vi "Robomapping.vi"(2 "Sensor View":i8[][](array[numeric]), 3 "World (mapped) in":i8[][](array[numeric]), 4 "Y":i8, 5 "X":i8) -> (0 "Sum of sensor array":i8, 1 "World (mapped) out":i8[][](array[numeric]))   [LabVIEW 2014]
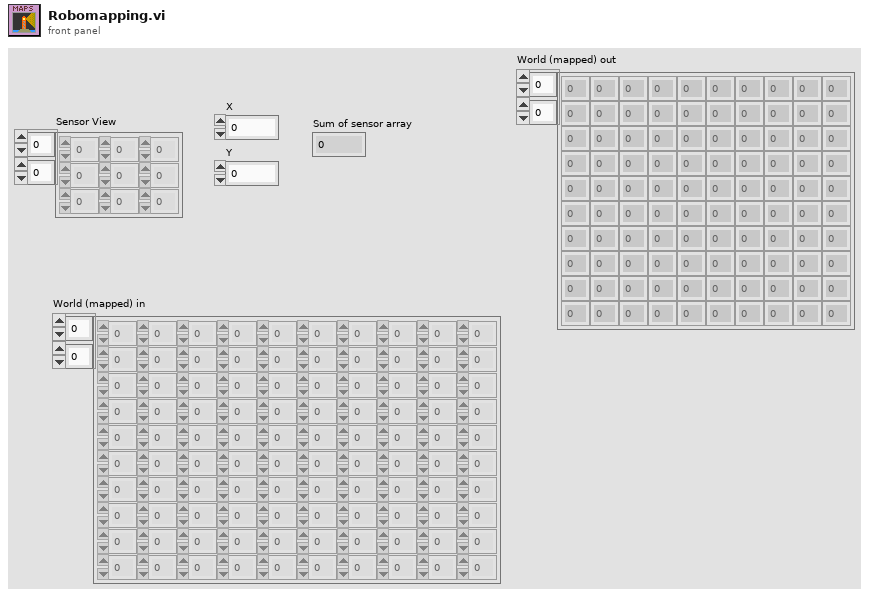
[diagram p1: front panel]
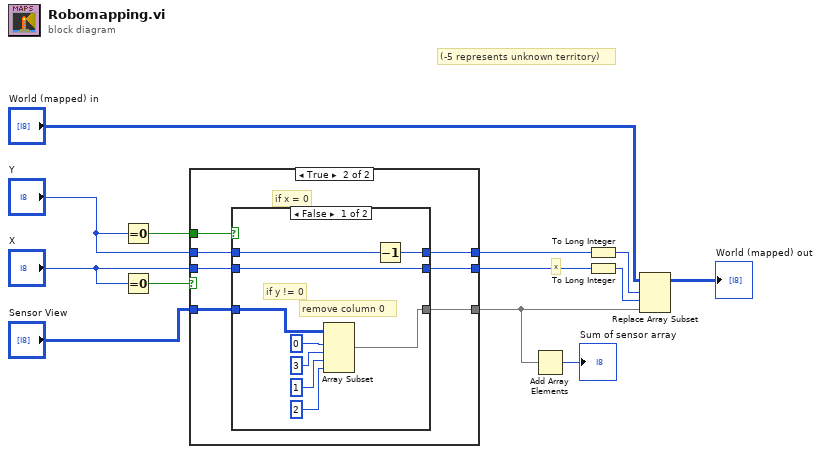
[diagram p0: block diagram]
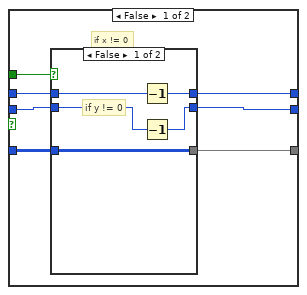
[diagram p2: hidden frame]
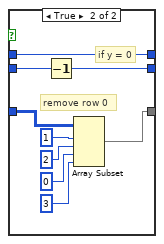
[diagram p3: hidden frame]
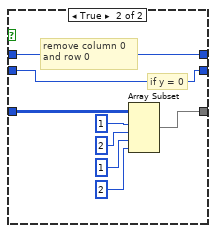
[diagram p4: hidden frame]
diagram:
  # "x"
  # "(-5 represents unknown territory)"
  n1 = Equal To 0?(x="Y") -> (x = 0?=w12:bool)
  n2 = Equal To 0?(x="X") -> (x = 0?=w13:bool)
  n3 = case shown="True" w13 {
    tunnel: "Sensor View" -> [w20 w40]
    tunnel: w12 -> [w19 w41]
    tunnel: [w16 w39] -> w2
    tunnel: "Y" -> [w18 w38]
    tunnel: [w17 w37] -> w11
    tunnel: "X" -> [w15 w36]
    tunnel: [w14 w35] -> w9
    frame False {
      # "if x != 0"
      n4 = case shown="False" w19 {
        tunnel: w20 -> [w25 w30]
        tunnel: w18 -> [w21 w26]
        tunnel: [w22 w26] -> w17
        tunnel: [w25 w29] -> w16
        tunnel: [w24 w27] -> w14
        tunnel: w15 -> [w23 w28]
        frame False {
          # "if y != 0"
          n5 = Decrement(x=w21) -> (x-1=w22:i8)
          n6 = Decrement(x=w23) -> (x-1=w24:i8)
        }
        frame True {
          # "remove row 0"
          # "if y = 0"
          n7 = Decrement(x=w28) -> (x-1=w27:i8)
          n8 = Array Subset(array=w30, index (row)=1 ("index"), length (row)=2 ("length"), index (col)=0 ("index"), length (col)=3 ("length")) -> (w29:i8[][])
        }
      }
    }
    frame True {
      # "if x = 0"
      n9 = case shown="False" w41 {
        tunnel: w40 -> [w46 w54]
        tunnel: [w45 w51] -> w39
        tunnel: w38 -> [w44 w52]
        tunnel: [w43 w52] -> w37
        tunnel: w36 -> [w42 w53]
        tunnel: [w42 w53] -> w35
        frame False {
          # "remove column 0"
          # "if y != 0"
          n10 = Array Subset(array=w46, index (row)=0 ("index"), length (row)=3 ("length"), index (col)=1 ("index"), length (col)=2 ("length")) -> (w45:i8[][])
          n11 = Decrement(x=w44) -> (x-1=w43:i8)
        }
        frame True {
          # "remove column 0\nand row 0"
          # "if y = 0"
          n12 = Array Subset(array=w54, index (row)=1 ("index"), length (row)=2 ("length"), index (col)=1 ("index"), length (col)=2 ("length")) -> (w51:i8[][])
        }
      }
    }
  }
  n13 = Add Array Elements(numeric array=w2) -> (sum=→"Sum of sensor array":i8)
  n14 = To Long Integer(number=w11) -> (32bit integer=w10:i32)
  n15 = To Long Integer(number=w9) -> (32bit integer=w8:i32)
  n16 = Replace Array Subset(array="World (mapped) in", new element=w2, index (row)=w10, index (col)=w8) -> (→"World (mapped) out":i8[][])
